vi "controlMode.vi"(7 "Set":bool, 8 "error in":errorcluster, 10 "Mode":i32, 11 "connection ID":refnum<k5>) -> (0 "error out":errorcluster, 2 "Mode out":i32, 3 "connection ID":refnum<k5>)   [LabVIEW 2016, in "AMC_VIs.lvlib"]
doc: "Gets the mode of RES application"
uses:
  AMC_VIs.lvlib
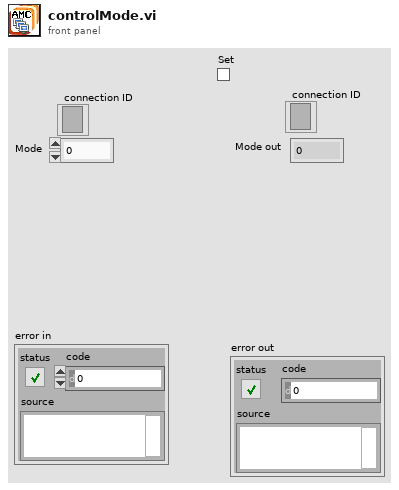
[diagram p1: front panel]
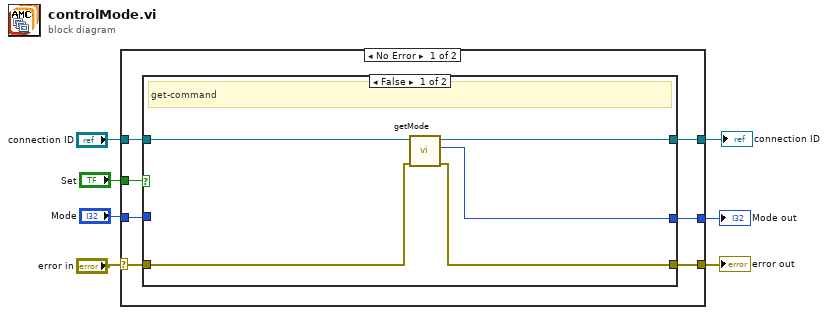
[diagram p0: block diagram]
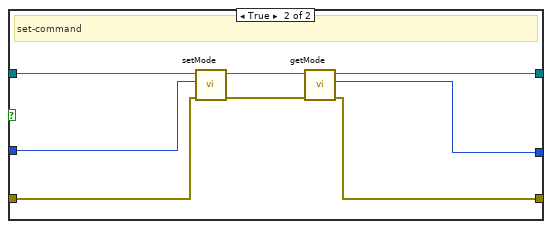
[diagram p2: hidden frame]
diagram:
  n1 = case shown="No Error" "error in" {
    selector: "error in" -> [w12 w28]
    tunnel: "Mode" -> [w14 w29]
    tunnel: [w11 w28] -> w6
    tunnel: "Set" -> [w13 _]
    tunnel: [w10 w29] -> w3
    tunnel: [w9 w30] -> w2
    tunnel: "connection ID" -> [w8 w30]
    frame No Error {
      n2 = case shown="False" w13 {
        tunnel: w14 -> [_ w22]
        tunnel: w12 -> [w16 w25]
        tunnel: [w17 w24] -> w11
        tunnel: [w15 w23] -> w10
        tunnel: [w18 w21] -> w9
        tunnel: w8 -> [w19 w20]
        frame False {
          # "get-command"
          n3 = call "getMode.vi"("error in"=w16, "connection ID"=w19) -> ("error out"=w17:errorcluster, "mode"=w15:i32, "connection ID"=w18:refnum<k5>)  [unwired: 7 in]
        }
        frame True {
          # "set-command"
          n4 = call "setMode.vi"("error in"=w25, "mode"=w22, "connection ID"=w20) -> ("error out"=w26:errorcluster, "connection ID"=w27:refnum<k5>)  [unwired: 7 in]
          n5 = call "getMode.vi"("error in"=w26, "connection ID"=w27) -> ("error out"=w24:errorcluster, "mode"=w23:i32, "connection ID"=w21:refnum<k5>)  [unwired: 7 in]
        }
      }
    }
    frame Error {
    }
  }
  "error out" <- w6
  "Mode out" <- w3
  "connection ID" <- w2
